vi "SEP_Hex.vi"(0 "System no.":i32=1 min=1 max=4 step=1, 2 "Axis to set":string[](array[string]), 3 "Parameter string":string[](array[string]), 4 "Password":string="100", 5 "error in":errorcluster, 6 "Parameter number (hex)":u32[](array[numeric]) format="%.0x") -> (14 "Controller error":bool, 19 "error out":errorcluster)   [LabVIEW 2026]
doc: "If password is correct, writes specified parameter values for specified hex. parameters of specified axes/channels to EPROM, waits 100 ms and queries ERR?. Controller error is TRUE if selected system reports an error code which is not 0. Old VI - please use SEP.vi instead.\n\nE-710: See E-710 GCS DLL Manual for a detailed list of available parameter numbers. Command is available in command level 1 only (see CCL.vi and CCL?.vi)\nE-761: See E-761 GCS DLL Manual for a detailed list of available parameter numbers."
panel:
  # "If password is correct, writes specified parameter values for specified hex. parameters of specified \naxes/channels to Eprom, waits 100 ms and queries ERR?. \nOld VI - please use SEP.vi instead."
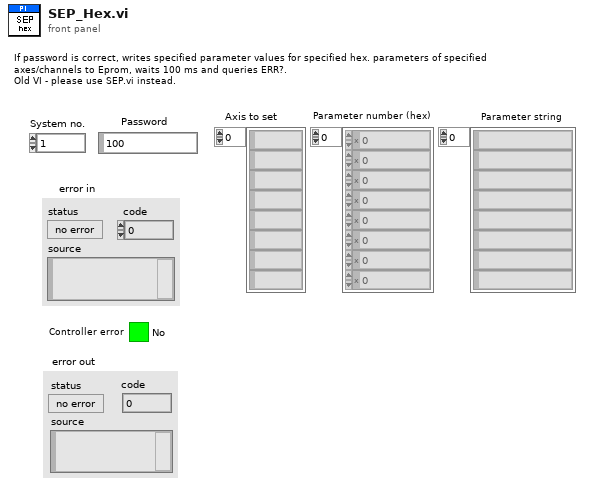
[diagram p1: front panel]
types:
  T1 = enum16{"Disable error check", "Force error check", "Use global settings"}
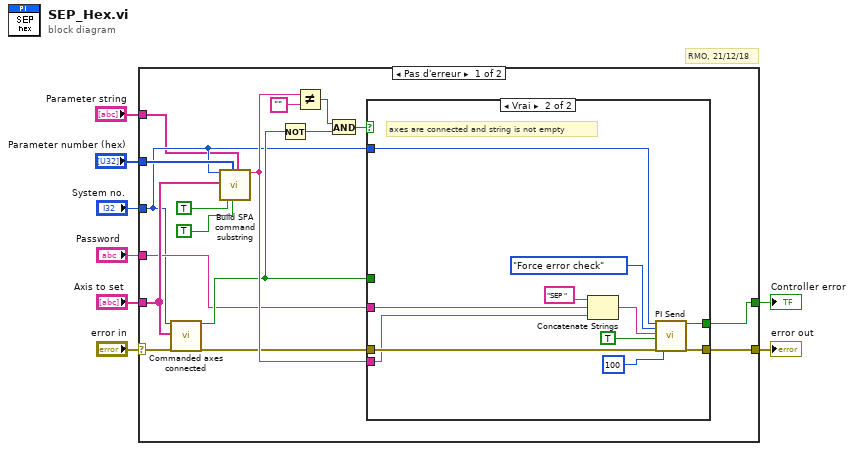
[diagram p0: block diagram]
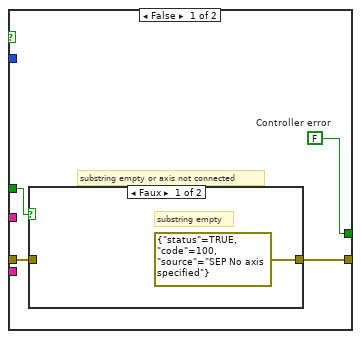
[diagram p2: hidden frame]
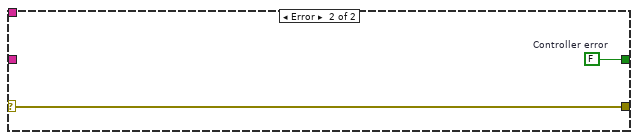
[diagram p4: hidden frame]
diagram:
  # "RMO, 21/12/18"
  n1 = case shown="Pas d'erreur" "error in" {
    selector: "error in" -> [w10 w44]
    tunnel: [w25 w44] -> w8
    tunnel: "Parameter string" -> [w13 _]
    tunnel: "System no." -> [w14 _]
    tunnel: "Axis to set" -> [w17 _]
    tunnel: "Parameter number (hex)" -> [w16 _]
    tunnel: "Password" -> [w15 _]
    tunnel: [w9 w43] -> w1
    frame No Error {
      n2 = call "Commanded axes connected.vi"("System no."=w14, "Commanded axes"=w17, "error in"=w10) -> ("Controller error"=w20:bool, "error out"=w22:errorcluster)  [unwired: 1 in, 14 out]
      n3 = call "Build SPA command substring.vi"("System no."=w14, "Axes to set"=w17, "Parameter no. format \n(Decimal: FALSE)"=TRUE ("Parameter no. format \n(Decimal: FALSE)"), "Parameter number (hex)"=w16, "Parameter format \n(Num.: FALSE)"=TRUE ("Parameter format \n(Num.: FALSE)"), "Parameter strings"=w13) -> ("SPA command substring"=w23:string)  [unwired: 4 in, 9 out]
      n4 = Not(x=w20) -> (.not. x?=w19:bool)
      n5 = Not Equal?(x=w23, y="") -> (x != y?=w21:bool)
      n6 = And(x=w21, y=w19) -> (x .and. y?=w18:bool)
      n7 = case shown="Vrai" w18 {
        tunnel: w23 -> [_ w37]
        tunnel: [w29 w34] -> w25
        tunnel: w22 -> [w27 w39]
        tunnel: w20 -> [w28 _]
        tunnel: w14 -> [_ w38]
        tunnel: w15 -> [_ w36]
        tunnel: [w26 w32] -> w9
        frame False {
          w26 = FALSE  # Controller error
          # "substring empty or axis not connected"
          n8 = case shown="Faux" w28 {
            tunnel: [errorcluster {"status"=TRUE, "code"=100, "source"="SEP No axis specified"} ("error out") w31] -> w29
            tunnel: w27 -> [_ w31]
            frame False {
              # "substring empty"
            }
            frame True {
              # "commanded axis not connected"
            }
          }
        }
        frame True {
          # "axes are connected and string is not empty"
          n9 = Concatenate Strings("SEP ", w36, w37) -> (w40:string)
          n10 = call "PI Send.vi"("System no."=w38, "Error check settings"=T1."Force error check", "String to send"=w40, "Attach termination char.?"=TRUE ("Attach Linefeed?"), "error in"=w39, "Delay before error check (ms)"=u32 100 ("milliseconds to wait")) -> ("Controller error"=w32:bool, "error out"=w34:errorcluster)  [unwired: 12 out]
        }
      }
    }
    frame Error {
      w43 = FALSE  # Controller error
    }
  }
  "error out" <- w8
  "Controller error" <- w1
